vi "CompPtSetup.vi"(0 "VISA IN":refnum<visa-resource-name>, 1 "Compression Pt.":enum16{".1", ".3", "1", "3"}(ring)=enum."1", 2 "CW Frq.":dbl=2000000000.0, 3 "Stop Power":i32=10, 4 "Start Power":i32=-20, 5 "error in":errorcluster, 6 "AVG?":bool=TRUE, 7 "Channel":i32=1, 8 "AVG":i32=20, 9 "Window":i32=1, 10 "Format":string(combo)="MLOGarithmic", 11 "Trace":i32=1, 13 "Filename":string="GainMag") -> (14 "VISA Out":refnum<visa-resource-name>, 15 "X Axis":dbl, 16 "Y Real":dbl, 19 "error out":errorcluster)   [LabVIEW 2018]
uses:
  PNA-X.lvlib
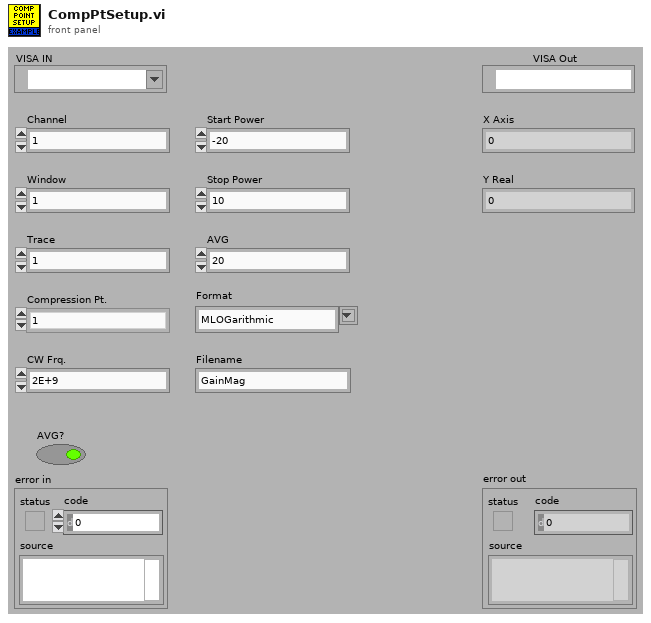
[diagram p1: front panel]
types:
  T1 = enum16{"All Off", "1", "2", "3", "4", "5", "6", "7", "8", "9", "Reference"}
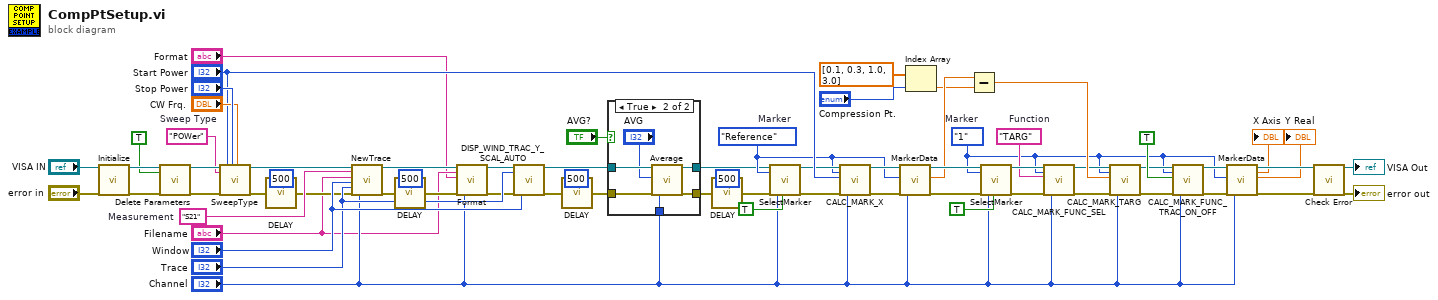
[diagram p0: block diagram]
diagram:
  w23 = "TARG"  # Function
  w21 = T1."1"  # Marker
  w22 = T1."Reference"  # Marker
  w50 = "S21"  # Measurement
  w54 = "POWer"  # Sweep Type
  n1 = call "Initialize.vi"("VISA IN"="VISA IN", "error in"="error in") -> ("VISA Out"=w67:refnum<visa-resource-name>, "error out"=w65:errorcluster)  [unwired: 15 in, 1 out]
  n2 = call "Delete Parameters .vi"("VISA IN"=w67, "Delete All?"=TRUE, "error in"=w65) -> ("VISA Out"=w57:refnum<visa-resource-name>, "error out"=w58:errorcluster)  [unwired: 15 in]
  n3 = call "SweepType.vi"("VISA IN"=w57, "Sweep Type"=w54, "error in"=w58, "Start Power"="Start Power", "Stop Power"="Stop Power", "CW Frq."="CW Frq.") -> ("VISA Out"=w52:refnum<visa-resource-name>, "error out"=w51:errorcluster)  [unwired: 12 in]
  n4 = call "DELAY.vi"("milliseconds to wait"=u32 500, "error in (no error)"=w51) -> ("error out"=w14:errorcluster)  [unwired: 13 in]
  n5 = call "NewTrace.vi"("VISA IN"=w52, "Measurement"=w50, "FileName"="Filename", "Window"="Window", "Trace"="Trace", "error in (no error)"=w14, "Channel"="Channel") -> ("VISA Out"=w7:refnum<visa-resource-name>, "error out"=w47:errorcluster)  [unwired: 11 in]
  n6 = call "DELAY.vi"("milliseconds to wait"=u32 500, "error in (no error)"=w47) -> ("error out"=w5:errorcluster)  [unwired: 13 in]
  n7 = call "Format.vi"("VISA IN"=w7, "Measurement Name"="Filename", "Format"="Format", "error in"=w5, "Channel"="Channel") -> ("VISA Out"=w6:refnum<visa-resource-name>, "error out"=w1:errorcluster)  [unwired: 13 in]
  n8 = call "DISP_WIND_TRAC_Y_SCAL_AUTO.vi"("VISA IN"=w6, "Trace"="Trace", "error in"=w1, "Window"="Window") -> ("VISA Out"=w46:refnum<visa-resource-name>, "error out"=w45:errorcluster)  [unwired: 14 in]
  n9 = call "DELAY.vi"("milliseconds to wait"=u32 500, "error in (no error)"=w45) -> ("error out"=w16:errorcluster)  [unwired: 13 in]
  n10 = case shown="True" "AVG?" {
    tunnel: "Channel" -> [_ w75]
    tunnel: w46 -> [w68 w74]
    tunnel: [w69 w72] -> w20
    tunnel: [w68 w71] -> w18
    tunnel: w16 -> [w69 w70]
    frame False {
    }
    frame True {
      n11 = call "Average.vi"("VISA IN"=w74, "AVG"="AVG", "error in"=w70, "Channel"=w75) -> ("VISA Out"=w71:refnum<visa-resource-name>, "error out"=w72:errorcluster)  [unwired: 14 in]
    }
  }
  n12 = call "DELAY.vi"("milliseconds to wait"=u32 500, "error in (no error)"=w20) -> ("error out"=w19:errorcluster)  [unwired: 13 in]
  n13 = call "SelectMarker.vi"("VISA IN"=w18, "Marker"=w22, "error in"=w19, "Channel"="Channel", "ON-OFF"=TRUE) -> ("VISA Out"=w35:refnum<visa-resource-name>, "error out"=w34:errorcluster)  [unwired: 13 in]
  n14 = call "CALC_MARK_X.vi"("VISA IN"=w35, "Marker number"=w22, "X-axis Position"="Start Power", "error in"=w34, "Channel"="Channel") -> ("VISA Out"=w32:refnum<visa-resource-name>, "error out"=w33:errorcluster)  [unwired: 13 in]
  n15 = call "MarkerData.vi"("VISA IN"=w32, "Marker number"=w22, "error in"=w33, "Channel"="Channel") -> ("VISA Out"=w43:refnum<visa-resource-name>, "Y Real"=w40:dbl, "error out"=w42:errorcluster)  [unwired: 11 in, 2 out]
  n16 = Index Array(array=dbl[] [0.1, 0.3, 1.0, 3.0], index="Compression Pt.") -> (element=w9:dbl)
  n17 = Subtract(x=w40, y=w9) -> (x-y=w38:dbl)
  n18 = call "SelectMarker.vi"("VISA IN"=w43, "Marker"=w21, "error in"=w42, "Channel"="Channel", "ON-OFF"=TRUE) -> ("VISA Out"=w27:refnum<visa-resource-name>, "error out"=w26:errorcluster)  [unwired: 13 in]
  n19 = call "CALC_MARK_FUNC_SEL.vi"("VISA IN"=w27, "Marker number"=w21, "Function"=w23, "error in"=w26, "Channel"="Channel") -> ("VISA Out"=w24:refnum<visa-resource-name>, "error out"=w25:errorcluster)  [unwired: 13 in]
  n20 = call "CALC_MARK_TARG.vi"("VISA IN"=w24, "Marker number"=w21, "Target Value"=w38, "error in"=w25, "Channel"="Channel") -> ("VISA Out"=w37:refnum<visa-resource-name>, "error out"=w36:errorcluster)  [unwired: 13 in]
  n21 = call "CALC_MARK_FUNC_TRAC_ON_OFF.vi"("VISA IN"=w37, "Marker number"=w21, "Track ON/OFF"=TRUE, "error in"=w36, "Channel"="Channel") -> ("VISA Out"=w31:refnum<visa-resource-name>, "error out"=w30:errorcluster)  [unwired: 13 in]
  n22 = call "MarkerData.vi"("VISA IN"=w31, "Marker number"=w21, "error in"=w30, "Channel"="Channel") -> ("VISA Out"=w61:refnum<visa-resource-name>, "X Axis"=→"X Axis":dbl, "Y Real"=→"Y Real":dbl, "error out"=w60:errorcluster)  [unwired: 11 in, 1 out]
  n23 = call "Check Error.vi"("VISA Resource Name"=w61, "error in (no error)"=w60) -> ("dup VISA session"=→"VISA Out":refnum<visa-resource-name>, "error out"=→"error out":errorcluster)  [unwired: 16 in]
